vi "Robot Global Data.vi"() -> ()   [LabVIEW 2012]
doc: "This global VI can contain as many global variables as you need. Place a control on the panel, give it a good name. To read or write to it from a VI, drag the icon to the diagram of that VI. You can also drag from the project. Click on the node to change which global you access. You shouldn't have multiple locations writing to a global or it will cause a race-condition."
uses:
  <vilib>/Rock Robotics/WPI/Camera/WPI_CameraImageSize.ctl
  <vilib>/Rock Robotics/WPI/DriverStation/WPI_DriverStationRobotMode2.ctl
panel:
  in  "Autonomous":bool
  in  "Left Ultrasonic Sensor":dbl(slide) scale=0.0..10.0
  in  "Reading Ultra":i32=1
  in  "Ultrasonic Scaling Factor (s/cm)":dbl=0.000147
  out "Running Config":bool
  in  "Arm Target Speed":dbl
  in  "Arm Target Pos":dbl
  out "Sending Arm to Target":bool
  in  "Hotkeys":dbl[][](array[numeric])
  in  "Right Ultrasonic Sensor":dbl(slide) scale=0.0..10.0
  out "Encoder Set":bool
  in  "Arm Output":dbl
  in  "X-Throttle":dbl(knob)=0.65 scale=0.0..1.0
  in  "Arm Encoder":dbl
  out "Simulator?":bool=TRUE
  in  "Y-Throttle":dbl(knob)=0.65 scale=0.0..1.0 scale format="%#_6f"
  out "Arm Motor Limit Override":bool
  out "Arm Limit":bool
  out "Arm Hook Sensor":bool
  in  "Robot Mode":T1
  in  "LED toggle rate (ms)":u32=20
  in  "image size":T2=enum."320x240"
  in  "Enable Vision":bool
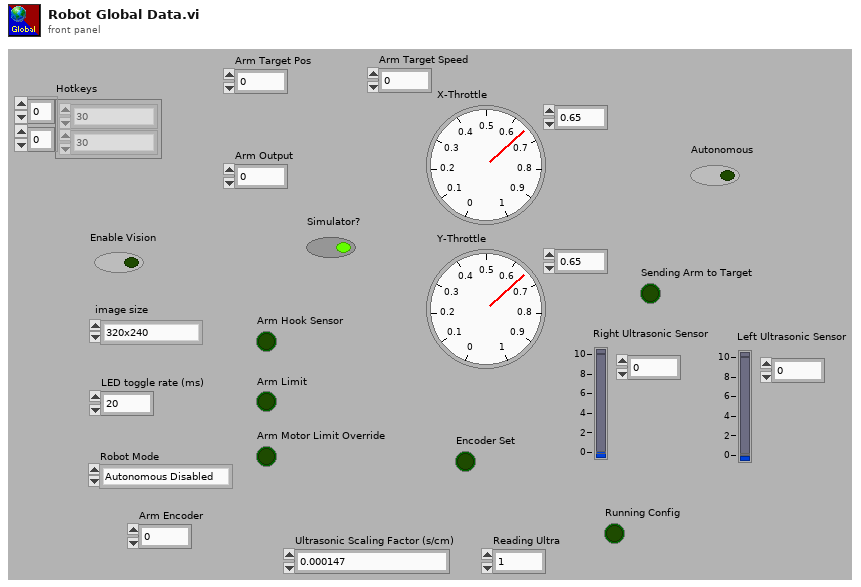
[diagram p1: front panel]
types:
  T1 = typedef "WPI_DriverStationRobotMode2.ctl" = enum16{"Autonomous Disabled", "Autonomous Enabled", "Teleop Disabled", "Teleop Enabled", "Timeout", "Finish", "Test Disabled", "Test Enabled"}
  T2 = typedef "WPI_CameraImageSize.ctl" = enum16{"640x480", "320x240", "160x120"}
diagram:
